vi "Intellirupter_sensor1.vi"() -> ()   [LabVIEW 2016]
uses:
  <vilib>/rvi/Emulation/niFpgaGetClockAttributes.vi
  <vilib>/rvi/Emulation/niFpgaSctlEmulationGetInTimedLoop.vi
  <vilib>/rvi/Emulation/niFpgaEmulationReportErrorSimple.vi
  <vilib>/rvi/eio/common/nirviEmuTemplateMethod_errors.vi
  <vilib>/rvi/interface/RandomDataEmulation/niFpgaRandomDataHandleErrors.vi
  <vilib>/rvi/Emulation/niFpgaCriticalErrorInLSC.vi
  <vilib>/eio/EIONode/EIONode.xnode
  <vilib>/rvi/DataTransferAndStorage/Container/XNode/niFpgaContainer.xnode
  <vilib>/rvi/interface/RandomDataEmulation/nirviRandomDataFpgaReadWriteTemplate.vi
panel:
  in  "Count(ticks)":u32=100
  out "Data FIFO Full":bool
  in  "Relay8":bool
  in  "Relay7":bool
  in  "Relay6":bool
  in  "Relay5":bool
  in  "Relay4":bool
  in  "Relay3":bool
  in  "Relay2":bool
  in  "Relay1":bool
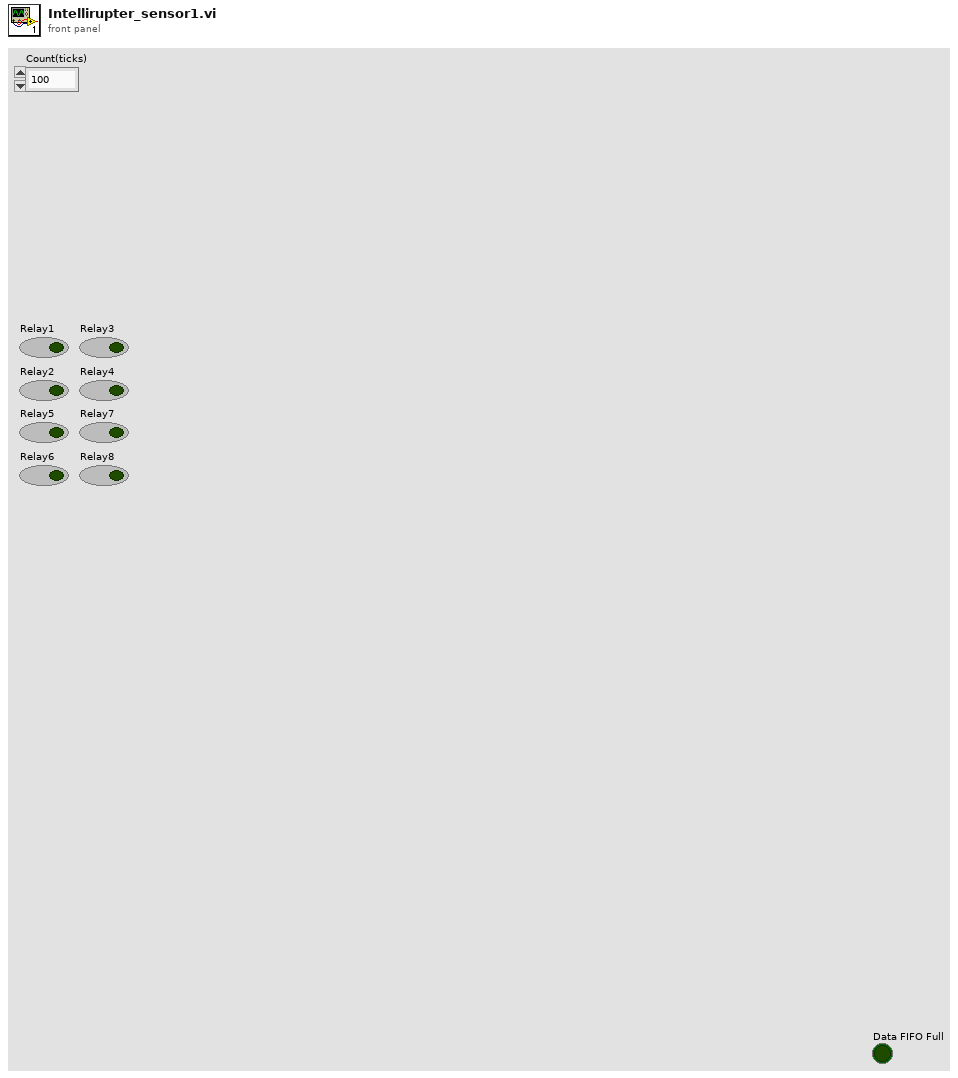
[diagram p1: front panel]
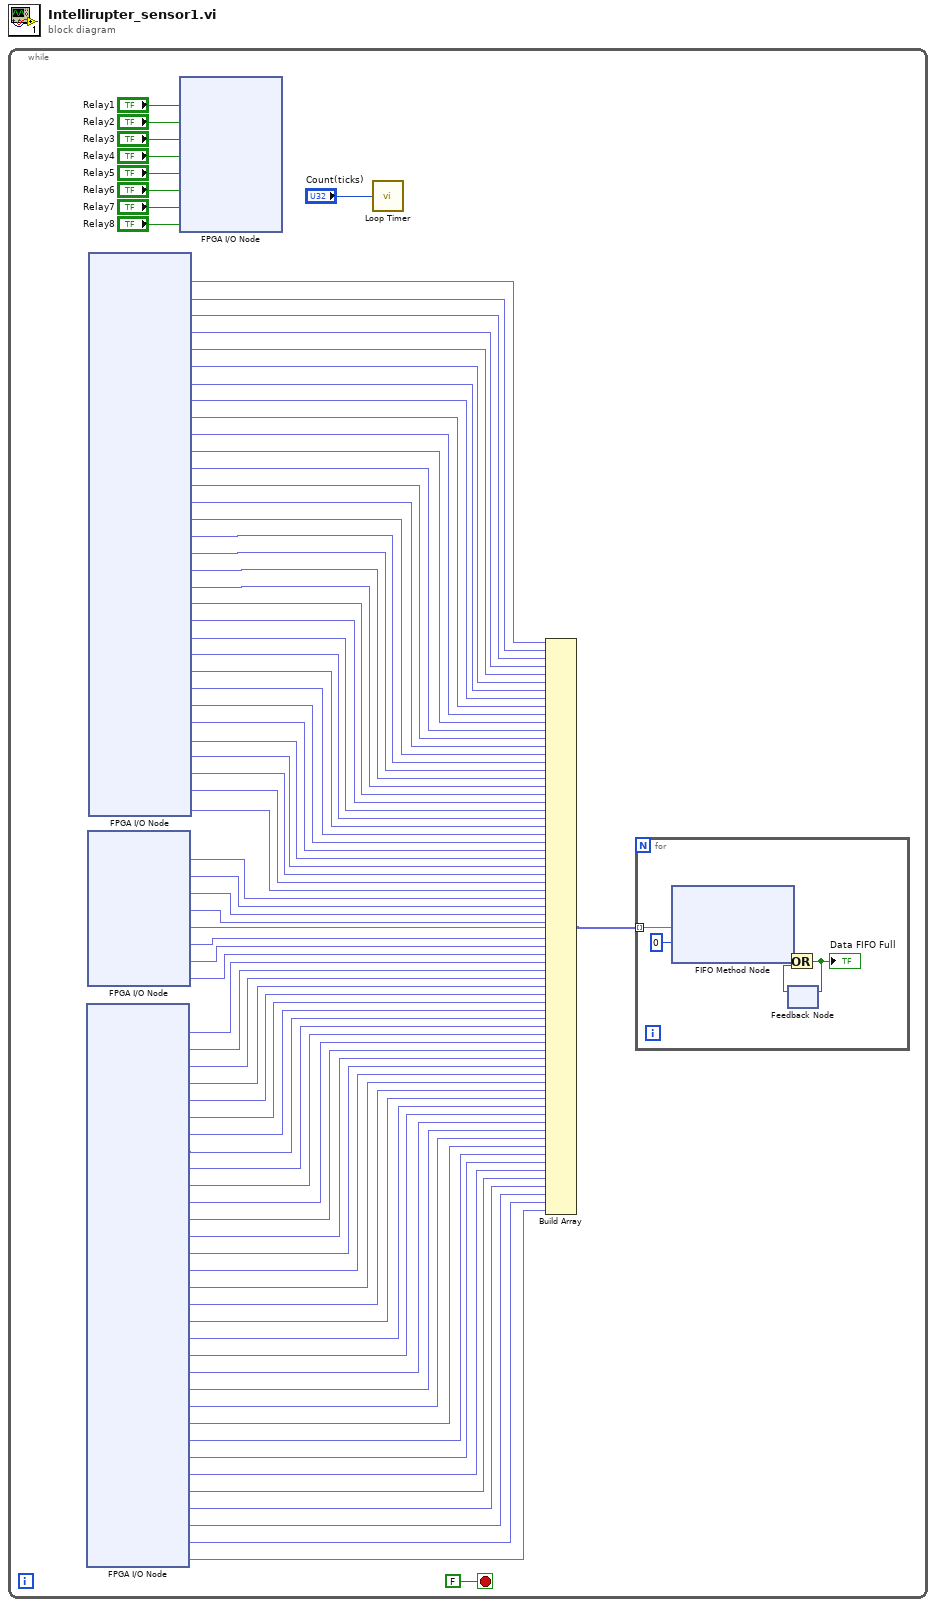
[diagram p0: block diagram]
diagram:
  n1 = while {
    stop <- FALSE stop-if-true
    n2 = xnode "FPGA I/O Node"() -> ("Mod7/AI0"=w42:fxp<+/-,26,5>, "Mod7/AI1"=w31:fxp<+/-,26,5>, "Mod7/AI2"=w30:fxp<+/-,26,5>, "Mod7/AI3"=w29:fxp<+/-,26,5>, "Mod7/AI4"=w28:fxp<+/-,26,5>, "Mod7/AI5"=w27:fxp<+/-,26,5>, "Mod7/AI6"=w26:fxp<+/-,26,5>, "Mod7/AI7"=w25:fxp<+/-,26,5>, "Mod7/AI8"=w24:fxp<+/-,26,5>, "Mod7/AI9"=w23:fxp<+/-,26,5>, "Mod7/AI10"=w22:fxp<+/-,26,5>, "Mod7/AI11"=w21:fxp<+/-,26,5>, "Mod7/AI12"=w20:fxp<+/-,26,5>, "Mod7/AI13"=w19:fxp<+/-,26,5>, "Mod7/AI14"=w1:fxp<+/-,26,5>, "Mod7/AI15"=w2:fxp<+/-,26,5>, "Mod7/AI16"=w3:fxp<+/-,26,5>, "Mod7/AI17"=w4:fxp<+/-,26,5>, "Mod7/AI18"=w5:fxp<+/-,26,5>, "Mod7/AI19"=w6:fxp<+/-,26,5>, "Mod7/AI20"=w7:fxp<+/-,26,5>, "Mod7/AI21"=w8:fxp<+/-,26,5>, "Mod7/AI22"=w9:fxp<+/-,26,5>, "Mod7/AI23"=w10:fxp<+/-,26,5>, "Mod7/AI24"=w11:fxp<+/-,26,5>, "Mod7/AI25"=w12:fxp<+/-,26,5>, "Mod7/AI26"=w13:fxp<+/-,26,5>, "Mod7/AI27"=w14:fxp<+/-,26,5>, "Mod7/AI28"=w15:fxp<+/-,26,5>, "Mod7/AI29"=w16:fxp<+/-,26,5>, "Mod7/AI30"=w17:fxp<+/-,26,5>, "Mod7/AI31"=w18:fxp<+/-,26,5>)  [unwired: 32 in, 32 out]
    n3 = xnode "FPGA I/O Node"() -> ("Mod5/AI20"=w50:fxp<+/-,26,5>, "Mod5/AI1"=w49:fxp<+/-,26,5>, "Mod5/AI2"=w48:fxp<+/-,26,5>, "Mod5/AI3"=w47:fxp<+/-,26,5>, "Mod5/AI0"=w46:fxp<+/-,26,5>, "Mod5/AI21"=w45:fxp<+/-,26,5>, "Mod5/AI22"=w44:fxp<+/-,26,5>, "Mod5/AI23"=w43:fxp<+/-,26,5>)  [unwired: 8 in, 8 out]
    n4 = xnode "FPGA I/O Node"() -> ("Mod1/AI0"=w82:fxp<+/-,26,5>, "Mod1/AI1"=w81:fxp<+/-,26,5>, "Mod1/AI2"=w80:fxp<+/-,26,5>, "Mod1/AI3"=w79:fxp<+/-,26,5>, "Mod1/AI4"=w78:fxp<+/-,26,5>, "Mod1/AI5"=w77:fxp<+/-,26,5>, "Mod1/AI6"=w76:fxp<+/-,26,5>, "Mod1/AI7"=w75:fxp<+/-,26,5>, "Mod1/AI8"=w74:fxp<+/-,26,5>, "Mod1/AI9"=w73:fxp<+/-,26,5>, "Mod1/AI10"=w72:fxp<+/-,26,5>, "Mod1/AI11"=w71:fxp<+/-,26,5>, "Mod1/AI12"=w70:fxp<+/-,26,5>, "Mod1/AI13"=w69:fxp<+/-,26,5>, "Mod1/AI14"=w68:fxp<+/-,26,5>, "Mod1/AI15"=w67:fxp<+/-,26,5>, "Mod1/AI16"=w66:fxp<+/-,26,5>, "Mod1/AI17"=w65:fxp<+/-,26,5>, "Mod1/AI18"=w64:fxp<+/-,26,5>, "Mod1/AI19"=w63:fxp<+/-,26,5>, "Mod1/AI20"=w62:fxp<+/-,26,5>, "Mod1/AI21"=w61:fxp<+/-,26,5>, "Mod1/AI22"=w60:fxp<+/-,26,5>, "Mod1/AI23"=w59:fxp<+/-,26,5>, "Mod1/AI24"=w58:fxp<+/-,26,5>, "Mod1/AI25"=w57:fxp<+/-,26,5>, "Mod1/AI26"=w56:fxp<+/-,26,5>, "Mod1/AI27"=w55:fxp<+/-,26,5>, "Mod1/AI28"=w54:fxp<+/-,26,5>, "Mod1/AI29"=w53:fxp<+/-,26,5>, "Mod1/AI30"=w52:fxp<+/-,26,5>, "Mod1/AI31"=w51:fxp<+/-,26,5>)  [unwired: 32 in, 32 out]
    n5 = xnode "FPGA I/O Node"("Mod6/DO0"="Relay1", "Mod6/DO1"="Relay2", "Mod6/DO2"="Relay3", "Mod6/DO3"="Relay4", "Mod6/DO4"="Relay5", "Mod6/DO5"="Relay6", "Mod6/DO6"="Relay7", "Mod6/DO7"="Relay8") -> ()  [unwired: 8 in, 8 out]
    n6 = call "Loop Timer"("Count(Ticks)"="Count(ticks)") -> ()  [unwired: 1 out]
    n7 = Build Array(w82, w81, w80, w79, w78, w77, w76, w75, w74, w73, w72, w71, w70, w69, w68, w67, w66, w65, w64, w63, w62, w61, w60, w59, w58, w57, w56, w55, w54, w53, w52, w51, w50, w49, w48, w47, w46, w45, w44, w43, w42, w31, w30, w29, w28, w27, w26, w25, w24, w23, w22, w21, w20, w19, w1, w2, w3, w4, w5, w6, w7, w8, w9, w10, w11, w12, w13, w14, w15, w16, w17, w18) -> (w40:fxp<+/-,26,5>[])
    n8 = for {
      tunnel: w40 -> [w84] mode=indexing
      n9 = xnode ("FIFO Method Node")("Element"=w84, "Timeout"=0) -> ("Timed Out?"=w86:bool)  [unwired: 1 in, 1 out]
      n10 = feedback #1() -> (w85:bool)  [unwired: 1 out]
      n11 = Or(x=w86, y=w85) -> (x .or. y?=w87:bool)
      "Data FIFO Full" <- w87
      n12 = feedback-in #1(w87) -> ()
    }
  }
